vi "DrawLine send pixel to fpga.vi"(6 "Color":u16, 7 "steep":bool, 8 "error in":errorcluster, 9 "X":i32, 10 "Y":i16, 11 "Refnum in":T1) -> (0 "error out":errorcluster, 3 "Refnum out":T1)   [LabVIEW 2019]
uses:
  TypeDefs/FPGA Reference.ctl
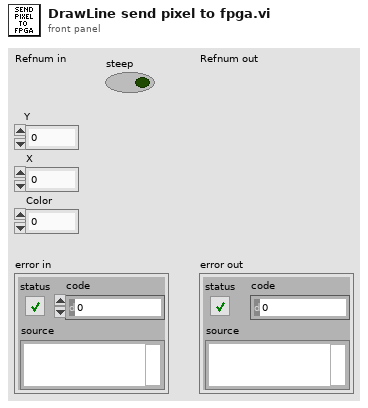
[diagram p1: front panel]
types:
  T1 = typedef "FPGA Reference.ctl" = refnum<k20>
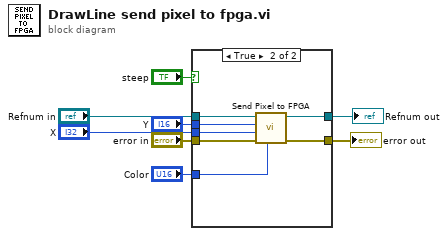
[diagram p0: block diagram]
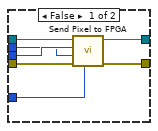
[diagram p2: hidden frame]
diagram:
  n1 = case shown="True" "steep" {
    tunnel: "X" -> [w15 w20]
    tunnel: "Y" -> [w14 w21]
    tunnel: "Color" -> [w13 w22]
    tunnel: "Refnum in" -> [w12 w19]
    tunnel: [w11 w18] -> w4
    tunnel: "error in" -> [w9 w17]
    tunnel: [w10 w16] -> w6
    frame False {
      n2 = call "Send Pixel to FPGA.vi"("Color"=w13, "error in"=w9, "Y"=w14, "X"=w15, "FPGA VI Reference Out"=w12) -> ("error out"=w10:errorcluster, "FPGA VI Reference Out 2"=w11:T1)  [unwired: 5 in]
    }
    frame True {
      n3 = call "Send Pixel to FPGA.vi"("Color"=w22, "error in"=w17, "Y"=w20, "X"=w21, "FPGA VI Reference Out"=w19) -> ("error out"=w16:errorcluster, "FPGA VI Reference Out 2"=w18:T1)  [unwired: 5 in]
    }
  }
  "error out" <- w6
  "Refnum out" <- w4
